vi "MGI Daemon.vi"(9 "Ignore Warnings? (F: Process Errors and Warnings)":bool, 10 "Error Log Directory":path, 11 "MGI Error Reporter Base In":refnum<class "MGI Error Reporter Base.lvclass">) -> (3 "MGI Error Reporter Base Out":refnum<class "MGI Error Reporter Base.lvclass">)   [LabVIEW 2020, in "MGI Error Reporter Base.lvclass"]
doc: "This Loop is called in a dynamically run VI and becomes the daemon for the Error Reporter. The MGI Error Reporter Base Daemon processes errors by logging them to file.\n\nAuthored by Shawn Walpole\nsupport@mooregoodideas.com\nwww.mooregoodideas.com\n\nCopyright (c) 2013, Moore Good Ideas, Inc.\n\nAll rights reserved.\n\nRedistribution and use in source and binary forms, with or without modification, are permitted provided that the following conditions are met:\n\n * Redistributions of source code must retain the above copyright notice, this list of conditions and the following disclaimer.\n * Redistributions in binary form must reproduce the above copyright notice, this list of conditions and the following disclaimer in the documentation and/or other materials provided with the distribution.\n * Neither the name of Moore Good Ideas, Inc. nor the names of its contributors may be used to endorse or promote products derived from this software without specific prior written permission.\n\nTHIS SOFTWARE IS PROVIDED BY THE COPYRIGHT HOLDERS AND CONTRIBUTORS \"AS IS\" AND ANY EXPRESS OR IMPLIED WARRANTIES, INCLUDING, BUT NOT LIMITED TO, THE IMPLIED WARRANTIES OF MERCHANTABILITY AND FITNESS FOR A PARTICULAR PURPOSE ARE DISCLAIMED. IN NO EVENT SHALL THE COPYRIGHT OWNER OR CONTRIBUTORS BE LIABLE FOR ANY DIRECT, INDIRECT, INCIDENTAL, SPECIAL, EXEMPLARY, OR CONSEQUENTIAL DAMAGES (INCLUDING, BUT NOT LIMITED TO, PROCUREMENT OF SUBSTITUTE GOODS OR SERVICES; LOSS OF USE, DATA, OR PROFITS; OR BUSINESS INTERRUPTION) HOWEVER CAUSED AND ON ANY THEORY OF LIABILITY, WHETHER IN CONTRACT, STRICT LIABILITY, OR TORT (INCLUDING NEGLIGENCE OR OTHERWISE) ARISING IN ANY WAY OUT OF THE USE OF THIS SOFTWARE, EVEN IF ADVISED OF THE POSSIBILITY OF SUCH DAMAGE."
uses:
  <userlib>/_MGI/Error Reporter/MGI Error Reporter Base/MGI Error Reporter Base.lvclass
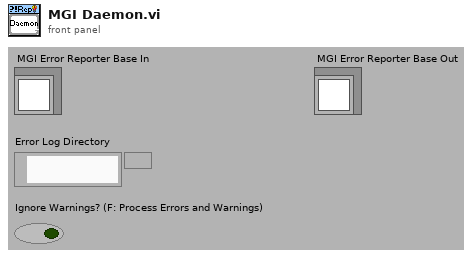
[diagram p1: front panel]
types:
  T1 = typedef "MGI Error Reporter Base.lvclass/Cmd Enum.ctl" = enum16{"Quit", "Show UI"}
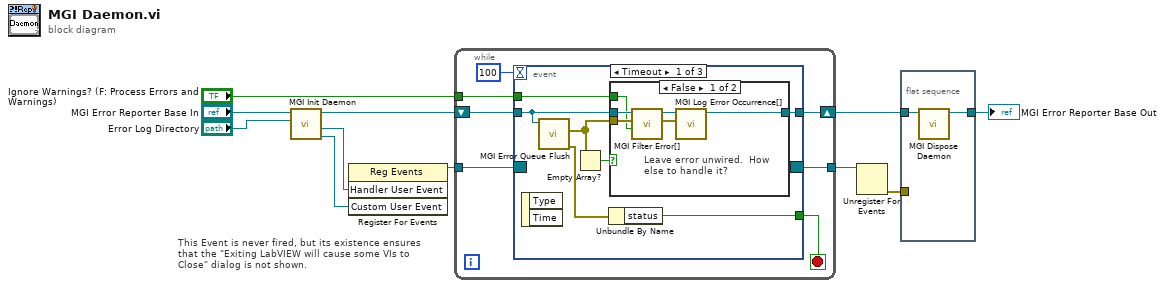
[diagram p0: block diagram]
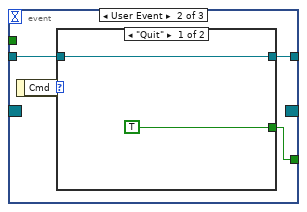
[diagram p3: hidden frame]
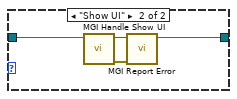
[diagram p4: hidden frame]
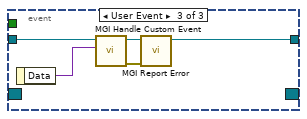
[diagram p5: hidden frame]
diagram:
  # "This Event is never fired, but its existence ensures that the \"Exiting LabVIEW will cause some VIs to Close\" dialog is not shown."
  n1 = call-dynamic "MGI Init Daemon.vi"("Err Dir"="Error Log Directory", "MGI Error Reporter Base In"="MGI Error Reporter Base In") -> ("Custom User Event"=w10:refnum<user-event>, "Handler User Event"=w11:refnum<user-event>, "MGI Error Reporter Base Out"=w9:refnum<class "MGI Error Reporter Base.lvclass">)  [unwired: 7 out]
  n2 = register-events(w11, w10) -> (reference out=w6:refnum<event-registration>)  [unwired: 2 in, 1 out]
  n3 = while {
    shift-right: [w15] -> w8
    shift-left: w9 -> [w18]
    tunnel: w6 -> [w17]
    tunnel: [w13] -> w5
    tunnel: "Ignore Warnings? (F: Process Errors and Warnings)" -> [w12]
    stop <- w14 stop-if-true
    n4 = event shown="[0] Timeout" {
      selector: w17 -> [_ _ _]
      dyn-events: [_ _ _] -> w13
      timeout: 100 -> [_ _ _]
      tunnel: w18 -> [w19 w34 w45]
      tunnel: [w24 w33 w44] -> w15
      tunnel: [w23 w36 _] -> w14
      tunnel: w12 -> [w22 _ _]
      event Timeout {
        n5 = event-data() -> ()  [unwired: 3 out]
        n6 = call-dynamic "MGI Error Queue Flush.vi"("MGI Error Reporter Base In"=w19) -> ("error out"=w20:errorcluster, "Error[]"=w21:errorcluster[])  [unwired: 1 in, 8 out]
        n7 = Empty Array?(array=w21) -> (empty?=w25:bool)
        n8 = Unbundle By Name(w20) -> ("status"=w23:bool)
        n9 = case shown="False" w25 {
          tunnel: w19 -> [w30 w32]
          tunnel: w21 -> [w28 _]
          tunnel: [w31 w32] -> w24
          tunnel: w22 -> [w26 _]
          frame False {
            # "Leave error unwired.  How else to handle it?"
            n10 = call-dynamic "MGI Filter Error[].vi"("Ignore Warnings? (F: Process Errors and Warnings)"=w26, "Error Occurence[]"=w28, "MGI Error Reporter Base in"=w30) -> ("Filtered Error[]"=w27:errorcluster[], "MGI Error Reporter Base out"=w29:refnum<class "MGI Error Reporter Base.lvclass">)  [unwired: 7 out]
            n11 = call-dynamic "MGI Log Error Occurrence[].vi"("Error Occurence[]"=w27, "MGI Error Reporter Base in"=w29) -> ("MGI Error Reporter Base out"=w31:refnum<class "MGI Error Reporter Base.lvclass">)  [unwired: 2 in, 7 out]
          }
          frame True {
          }
        }
      }
      event User Event {
        n12 = event-data() -> ("Cmd"=w35:T1)  [unwired: 1 out]
        n13 = case shown="\"Quit\"" w35 {
          tunnel: [TRUE _] -> w36
          tunnel: w34 -> [w38 w41]
          tunnel: [w38 w40] -> w33
          frame "Quit" {
          }
          frame "Show UI" {
            n14 = call-dynamic "MGI Handle Show UI.vi"("MGI Error Reporter Base In"=w41) -> ("error out"=w39:errorcluster, "MGI Error Reporter Base Out"=w40:refnum<class "MGI Error Reporter Base.lvclass">)  [unwired: 2 in, 7 out]
            n15 = call <userlib>:"MGI Report Error.vi"("error in"=w39) -> ()  [unwired: 11 out]
          }
        }
      }
      event User Event {
        n16 = event-data() -> ("Data"=w43:variant)  [unwired: 1 out]
        n17 = call-dynamic "MGI Handle Custom Event.vi"("Data"=w43, "MGI Error Reporter Base In"=w45) -> ("error out"=w42:errorcluster, "MGI Error Reporter Base In"=w44:refnum<class "MGI Error Reporter Base.lvclass">)  [unwired: 1 in, 7 out]
        n18 = call <userlib>:"MGI Report Error.vi"("error in"=w42) -> ()  [unwired: 11 out]
      }
    }
  }
  n19 = Unregister For Events(event registration refnum=w5) -> (error out=w4:errorcluster)  [unwired: 1 in]
  n20 = flat-sequence {
    tunnel: w8 -> [w47]
    tunnel: [w46] -> w7
    tunnel: w4 -> [_]
    frame #0 {
      n21 = call-dynamic "MGI Dispose Daemon.vi"("MGI Error Reporter Base In"=w47) -> ("MGI Error Reporter Base Out"=w46:refnum<class "MGI Error Reporter Base.lvclass">)  [unwired: 10 out]
    }
  }
  "MGI Error Reporter Base Out" <- w7
